vi "Display Text Test.vi"() -> ()   [LabVIEW 2019]
uses:
  Display/Public/Controls/Size.ctl
  String/String.lvclass
  C:/Users/goo13/Documents/GIT Local/myRIO-Neopixel/Source/RT/Display Element/Display Element.lvclass
  Display Element/Public/Controls/Vector.ctl
  Display/Display.lvclass
  Display Element/Display Element.lvclass
panel:
  in  "Text":string
  out "Frame":u32[][](array[colorbox])
  in  "stop":bool
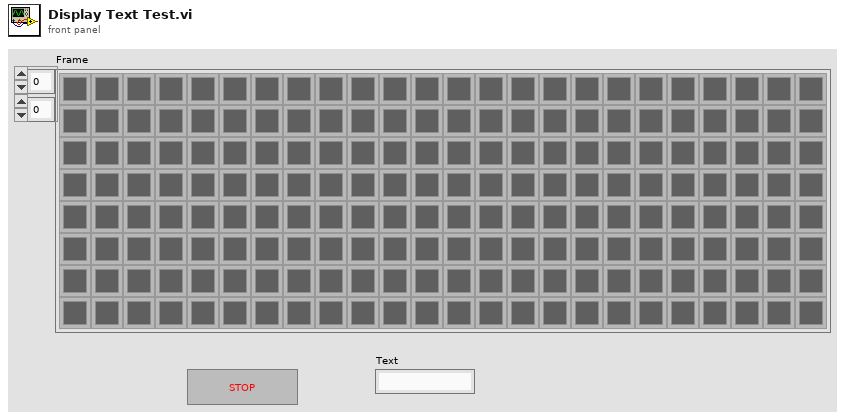
[diagram p1: front panel]
types:
  T1 = typedef "Display Element.lvclass/Vector.ctl" = cluster{"X":i32, "Y":i32}
  T2 = typedef "Display.lvclass/Size.ctl" = cluster{"Width":i32, "Height":i32}
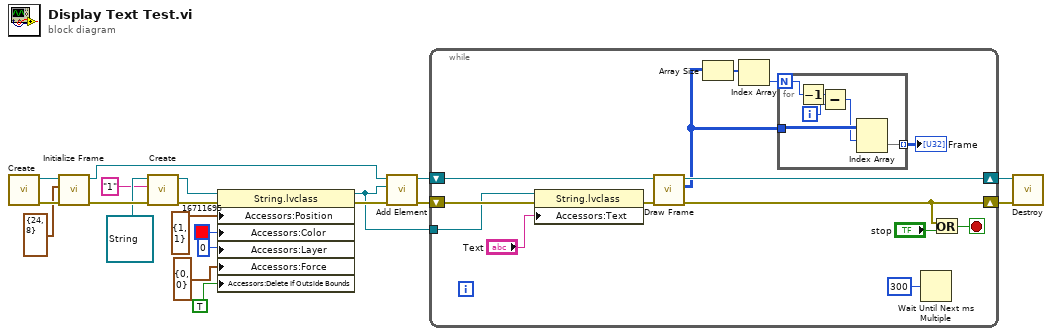
[diagram p0: block diagram]
diagram:
  n1 = call "Create.vi"() -> ("Error Out"=w17:errorcluster, "Screen Out"=w18:refnum<class "Display.lvclass">)  [unwired: 10 in]
  n2 = call "Initialize Frame.vi"("Error In"=w17, "Size"=T2 {"Width"=24, "Height"=8}, "Display In"=w18) -> ("Error Out"=w15:errorcluster, "Display Out"=w14:refnum<class "Display.lvclass">)  [unwired: 7 in]
  n3 = call-dynamic "Create.vi"("Error In"=w15, "Tag"="1", "Pixel In"=refnum<class "String.lvclass"> refnum ("String.lvclass")) -> ("Error Out"=w8:errorcluster, "Pixel Out"=w9:refnum<class "String.lvclass">)  [unwired: 7 in]
  n4 = property class="String.lvclass"(reference=w9, error in=w8, "Accessors:Position"=T1 {"X"=1, "Y"=1} ("Position"), "Accessors:Color"=u32 16711695 ("Color"), "Accessors:Layer"=u32 0 ("Layer"), "Accessors:Force"=T1 {"X"=0, "Y"=0} ("Force"), "Accessors:Delete If Outside Bounds"=TRUE ("Delete If Outside Bounds")) -> (reference out=w3:refnum<class "String.lvclass">, error out=w11:errorcluster)
  n5 = call "Add Element.vi"("Error In"=w11, "New Element"=w3, "Display In"=w14) -> ("Error Out"=w12:errorcluster, "Display Out"=w13:refnum<class "Display.lvclass">)  [unwired: 7 in]
  n6 = while {
    shift-right: [w32] -> w19
    shift-left: w12 -> [w26]
    shift-right: [w34] -> w20
    shift-left: w13 -> [w25]
    tunnel: w3 -> [w24]
    stop <- w30 stop-if-true
    n7 = property class="String.lvclass"(reference=w24, error in=w26, "Accessors:Text"="Text") -> (error out=w23:errorcluster)  [unwired: 1 out]
    n8 = call "Draw Frame.vi"("Error In"=w23, "Display In"=w25) -> ("Error Out"=w32:errorcluster, "Frame"=w21:u32[][], "Display Out"=w34:refnum<class "Display.lvclass">)  [unwired: 7 in]
    n9 = Array Size(array=w21) -> (size(s)=w29:i32[])
    n10 = Index Array(array=w29) -> (element=w28:i32)  [unwired: 1 in]
    n11 = for {
      N: w28 -> [w37]
      tunnel: w21 -> [w39]
      tunnel: [w35] -> w22 mode=indexing
      i -> [w40]
      n12 = Decrement(x=w37) -> (x-1=w36:i32)
      n13 = Subtract(x=w36, y=w40) -> (x-y=w38:i32)
      n14 = Index Array(array=w39, index (row)=w38) -> (element=w35:u32[])  [unwired: 1 in]
    }
    "Frame" <- w22
    n15 = Wait Until Next ms Multiple(millisecond multiple=u32 300) -> ()  [unwired: 1 out]
    n16 = Or(x=w32, y="stop") -> (x .or. y?=w30:bool)
  }
  n17 = call "Destroy.vi"("Error In"=w19, "Display In"=w20) -> ()  [unwired: 9 in, 1 out]
